vi "DbClicked Row.vi"(8 "错误输入（无错误）":errorcluster, 11 "Ref":refnum<vi>) -> (0 "错误输出":errorcluster, 2 "DbClicked Row":i32, 3 "Dup Ref":refnum<vi>)   [LabVIEW 2012, in "Mlistbox Tools.lvlib"]
uses:
  Mlistbox Tools.lvlib
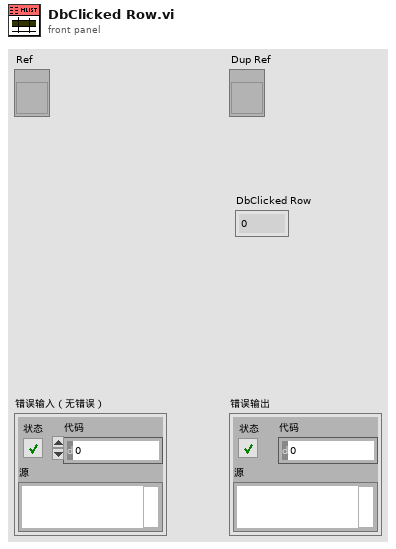
[diagram p1: front panel]
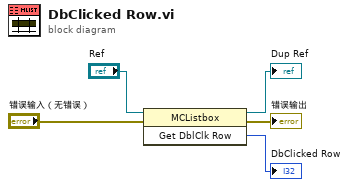
[diagram p0: block diagram]
diagram:
  n1 = invoke class="MCListbox" method="Get DblClk Row"(reference="Ref", error in="错误输入（无错误）") -> (reference out=→"Dup Ref":refnum<vi>, error out=→"错误输出":errorcluster, "Get Double-clicked Row"=→"DbClicked Row":i32)  [unwired: 1 in]
